vi "TelegramBOT_Create.vi"(0 "reference in":refnum<class "TelegramBOT.lvclass">, 2 "BOTToken(bot<token>)":string, 3 "AllowedSenders (empty = All)":string[](array[string]), 4 "AllowedMessages (empty = All)":string[](array[string]), 5 "error in (no error)":errorcluster) -> (14 "reference out":refnum<class "TelegramBOT.lvclass">, 19 "error out":errorcluster)   [LabVIEW 2019, in "TelegramBOT.lvclass"]
uses:
  TelegramBOT.lvclass
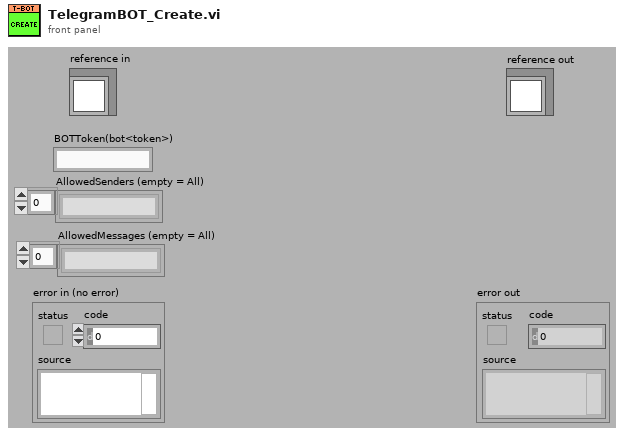
[diagram p1: front panel]
types:
  T1 = typedef "TelegramBOT.lvclass/ObjectAttributes.ctl" = cluster{"BOTToken":string, "AllowedSenders":string[], "AllowedMessages":string[]}
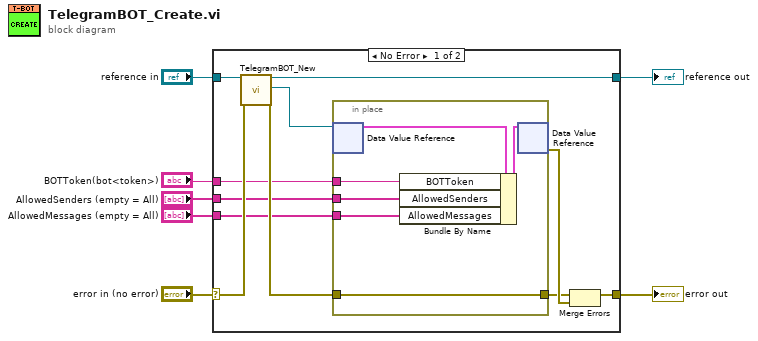
[diagram p0: block diagram]
diagram:
  n1 = case shown="No Error" "error in (no error)" {
    selector: "error in (no error)" -> [w17 w26]
    tunnel: [w14 w26] -> w6
    tunnel: "reference in" -> [w18 w25]
    tunnel: [w16 w25] -> w4
    tunnel: "BOTToken(bot<token>)" -> [w10 _]
    tunnel: "AllowedMessages (empty = All)" -> [w9 _]
    tunnel: "AllowedSenders (empty = All)" -> [w8 _]
    frame No Error {
      n2 = call "TelegramBOT_New.vi"("reference in"=w18, "error in (no error)"=w17) -> ("reference out"=w16:refnum<class "TelegramBOT.lvclass">, "DVRRefOut"=w13:refnum<data-value>, "error out"=w12:errorcluster)  [unwired: 14 in, 1 out]
      n3 = in-place {
        in-place-border: w12 -> [w22]
        in-place-border: [w22] -> w11
        in-place-border: w10 -> [w21]
        in-place-border: w9 -> [w20]
        in-place-border: w8 -> [w19]
        n4 = in-place-dvr #1(w13) -> (w23:T1)  [unwired: 1 out]
        n5 = Bundle By Name(cluster=w23, "BOTToken"=w21, "AllowedSenders"=w19, "AllowedMessages"=w20) -> (w24:T1)
        n6 = in-place-dvr #1(w24) -> (w15:errorcluster)  [unwired: 1 out]
      }
      n7 = Merge Errors(w11, w15) -> (w14:errorcluster)
    }
    frame Error {
      # "VI-TechBaseTemplate_Simple_6x8x6"
    }
  }
  "error out" <- w6
  "reference out" <- w4
